vi "Read waveplate in position.vi"(8 "error in (no error)":errorcluster, 11 "Sim_Ixon_Ultra in":refnum<class "Sim_Ixon_Ultra.lvclass">) -> (0 "error out":errorcluster, 2 "waveplate in position":bool, 3 "Sim_Ixon_Ultra out":refnum<class "Sim_Ixon_Ultra.lvclass">)   [LabVIEW 2018, in "Sim_Ixon_Ultra.lvclass"]
uses:
  Sim_Ixon_Ultra.lvclass
  Sim_Ixon_Ultra.lvclass/Sim_Ixon_Ultra.ctl
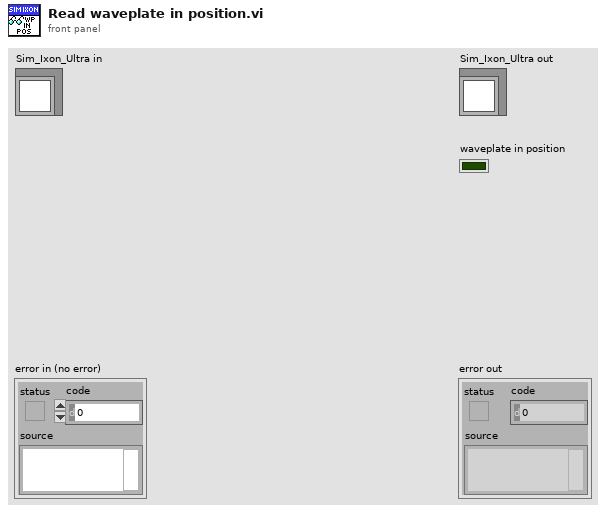
[diagram p1: front panel]
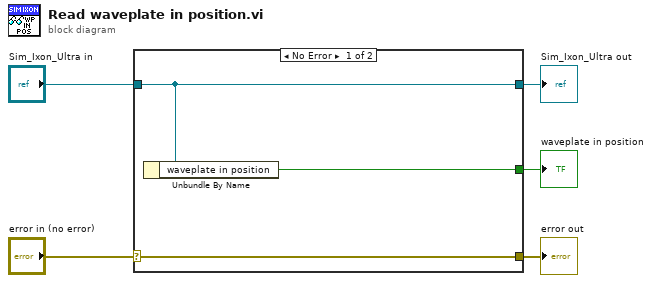
[diagram p0: block diagram]
diagram:
  n1 = case shown="No Error" "error in (no error)" {
    selector: "error in (no error)" -> [w8 w9]
    tunnel: [w8 w9] -> w4
    tunnel: [w7 w10] -> w2
    tunnel: "Sim_Ixon_Ultra in" -> [w7 w10]
    tunnel: [w6 _] -> w1
    frame No Error {
      n2 = Unbundle By Name(w7) -> ("waveplate in position"=w6:bool)
    }
    frame Error {
    }
  }
  "error out" <- w4
  "Sim_Ixon_Ultra out" <- w2
  "waveplate in position" <- w1
